vi "Disconnect All.vi"(8 "error in (no error)":errorcluster, 11 "Mock NI-SWITCH Consumer in":refnum<class "Mock NI-SWITCH Consumer.lvclass">=refnum) -> (0 "error out":errorcluster, 3 "Mock NI-SWITCH Consumer out":refnum<class "Mock NI-SWITCH Consumer.lvclass">)   [LabVIEW 2017, in "Mock NI-SWITCH Consumer.lvclass"]
uses:
  Mock NI-SWITCH Consumer.lvclass
  Mock NI-SWITCH Consumer.lvclass/Mock NI-SWITCH Consumer.ctl
  NI-SWITCH Consumer/NI-SWITCH Consumer.lvclass
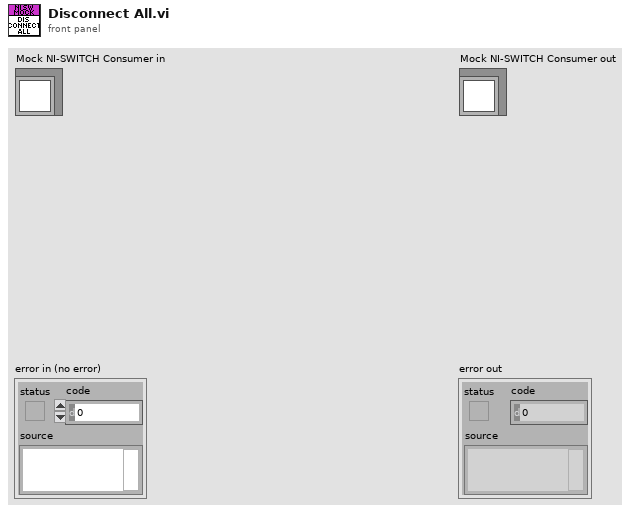
[diagram p1: front panel]
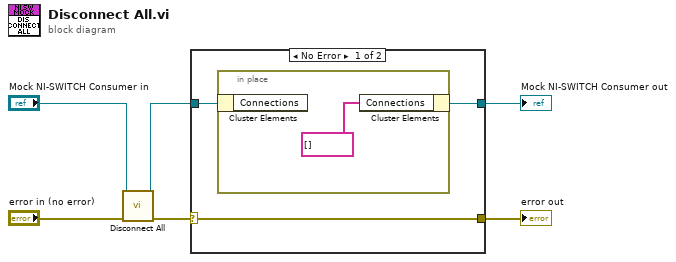
[diagram p0: block diagram]
diagram:
  n1 = call-parent "Disconnect All.vi"("error in (no error)"="error in (no error)", "SLSC Switch Consumer in"="Mock NI-SWITCH Consumer in") -> ("error out"=w4:errorcluster, "SLSC Switch Consumer out"=w3:refnum<class "Mock NI-SWITCH Consumer.lvclass">)  [unwired: 8 in]
  n2 = case shown="No Error" w4 {
    selector: w4 -> [w7 w11]
    tunnel: w3 -> [w9 w12]
    tunnel: [w8 w12] -> w2
    tunnel: [w7 w11] -> w1
    frame No Error {
      n3 = in-place {
        n4 = in-place-cluster #1(w9) -> ()  [unwired: 1 out]
        n5 = in-place-cluster #1("Connections"=string[] []) -> (w8:refnum<class "Mock NI-SWITCH Consumer.lvclass">)
      }
    }
    frame Error {
    }
  }
  "error out" <- w1
  "Mock NI-SWITCH Consumer out" <- w2
